vi "TEST_TRAJECTORY_EXECUTE_SWERVE.vi"(6 "EnableClosedLoop":bool=TRUE, 7 "Orientation Dmd In":dbl, 8 "Init":bool=TRUE, 9 "Reverse":bool, 10 "Follow Orientation":bool) -> (0 "AtReference":bool, 3 "Chassis Velocity Target":T2 {"vOmega" format="%10.3f"; "vY" format="%10.3f"; "vX" format="%10.3f"}, 4 "Time Offset":dbl=-1.0 format="%16.4f", 5 "Orientation Target":dbl, 11 "Gyro Heading":dbl)   [LabVIEW 2020]
uses:
  Robot Global Data.vi
  <vilib>/Rock Robotics/WPI/ThirdParty/JAS_Junk/TrajLib/Trajectory_Library.lvlib
  <vilib>/Rock Robotics/WPI/ThirdParty/JAS_Junk/TrajLib/TypeDef/CHASSIS_SPEEDS.ctl
  <vilib>/Rock Robotics/WPI/ThirdParty/JAS_Junk/TrajLib/TypeDef/TRANSLATION2D.ctl
  <vilib>/Rock Robotics/WPI/ThirdParty/JAS_Junk/TrajLib/TypeDef/ROTATION2D.ctl
  <vilib>/Rock Robotics/WPI/ThirdParty/JAS_Junk/TrajLib/TypeDef/POSE2D.ctl
  <vilib>/Rock Robotics/WPI/ThirdParty/JAS_Junk/TrajLib/TypeDef/TRAJ_STATE.ctl
panel:
  in  "Tab Control":T1(tab)
  out "OutputTRAJ_STATE":T3={"TimeSeconds"=0.0, "Velocity"=0.0, "Acceleration"=0.0, "POSE"={"TRANSLATION"={"X"=0.0, "Y"=0.0}, "ROTATION"={"VALUE"=0.0, "COS"=1.0, "SIN"=0.0}}, "Curvature"=0.0} {"POSE"."ROTATION"."SIN" format="%13.4f"; "POSE"."ROTATION"."COS" format="%13.4f"; "POSE"."ROTATION"."VALUE" format="%13.4f"; "POSE"."TRANSLATION"."Y" format="%14.3f"; "POSE"."TRANSLATION"."X" format="%14.3f"}
  in  "Step":bool
  in  "Trajectory File Name":path=path "Sample-Robot-2-Trajectory-TrajLibrary.csv"
  out "Traj File Good":bool
  out "Module Ang\nRadians":dbl
  out "Module Speed\nM/S":dbl
  in  "Run":bool
  out "Rel Odom":T4={"TRANSLATION"={"X"=0.0, "Y"=0.0}, "ROTATION"={"VALUE"=0.0, "COS"=1.0, "SIN"=0.0}} {"ROTATION"."SIN" format="%13.4f"; "ROTATION"."COS" format="%13.4f"; "ROTATION"."VALUE" format="%13.4f"; "TRANSLATION"."Y" format="%14.3f"; "TRANSLATION"."X" format="%14.3f"}
  out "Error and Corr":T7 {"Error Pose"."ROTATION"."SIN" format="%13.4f"; "Error Pose"."ROTATION"."COS" format="%13.4f"; "Error Pose"."ROTATION"."VALUE" format="%13.4f"; "Error Pose"."TRANSLATION"."Y" format="%14.3f"; "Error Pose"."TRANSLATION"."X" format="%14.3f"}
  out "Abs Odom":T4={"TRANSLATION"={"X"=0.0, "Y"=0.0}, "ROTATION"={"VALUE"=0.0, "COS"=1.0, "SIN"=0.0}} {"ROTATION"."SIN" format="%13.4f"; "ROTATION"."COS" format="%13.4f"; "ROTATION"."VALUE" format="%13.4f"; "TRANSLATION"."Y" format="%14.3f"; "TRANSLATION"."X" format="%14.3f"}
  out "Traj Err":cluster{"X":dbl, "Y":dbl, "Angle":dbl}(graph)
  out "Traj Correction":cluster{"X Corr":dbl, "Y Corr":dbl}(graph)
  out "Robot Position":cluster{dbl[], dbl[]}(graph)
  # "Module States"
  # "For now all modules use this value..."
  # "(FOR TESTING)"
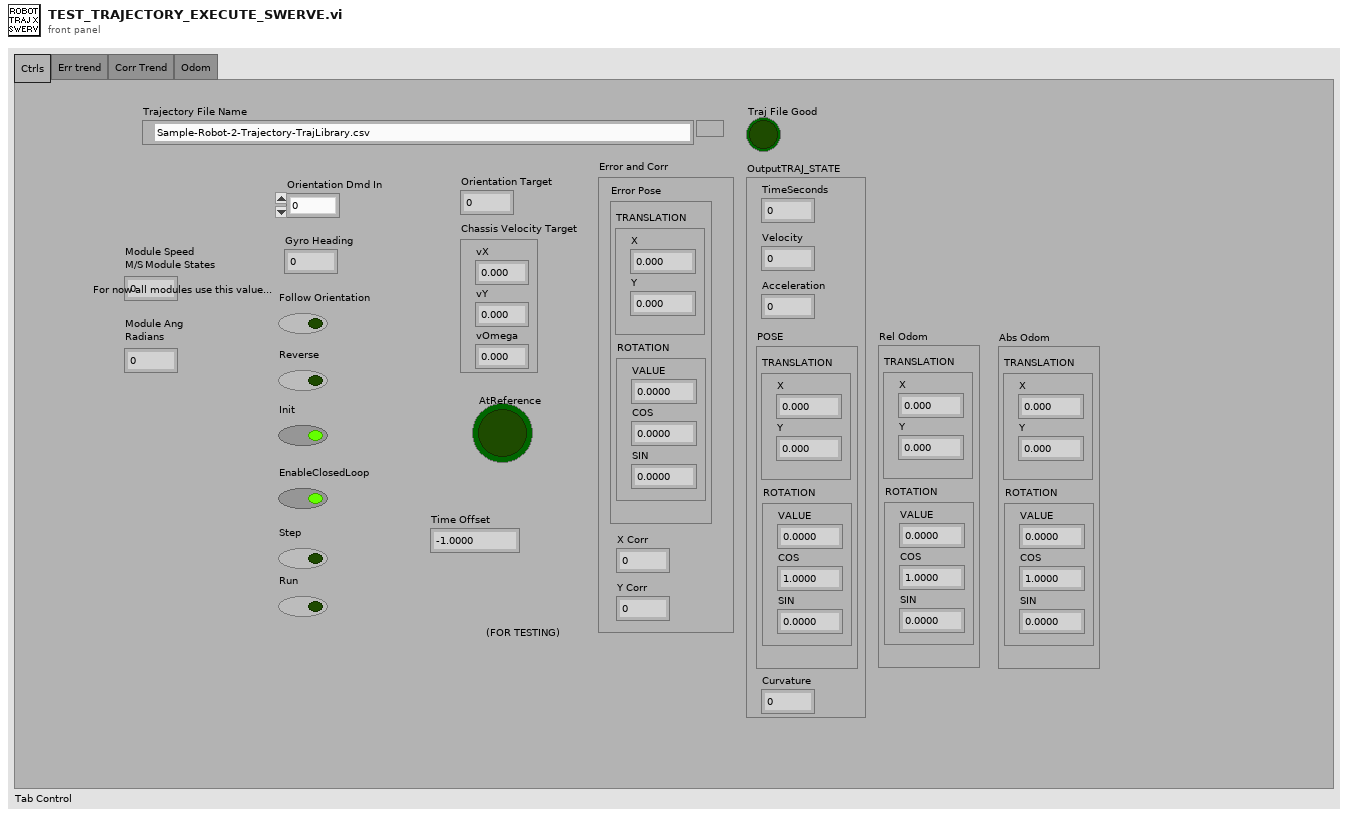
[diagram p1: front panel]
types:
  T1 = enum32{"Ctrls", "Err trend", "Corr Trend", "Odom"}
  T2 = typedef "Trajectory_Library.lvlib/CHASSIS_SPEEDS.ctl" = cluster{"vX":dbl, "vY":dbl, "vOmega":dbl}
  T3 = typedef "Trajectory_Library.lvlib/TRAJ_STATE.ctl" = cluster{"TimeSeconds":dbl, "Velocity":dbl, "Acceleration":dbl, "POSE":T4, "Curvature":dbl}
  T4 = typedef "Trajectory_Library.lvlib/POSE2D.ctl" = cluster{"TRANSLATION":T5, "ROTATION":T6}
  T5 = typedef "Trajectory_Library.lvlib/TRANSLATION2D.ctl" = cluster{"X":dbl, "Y":dbl}
  T6 = typedef "Trajectory_Library.lvlib/ROTATION2D.ctl" = cluster{"VALUE":dbl, "COS":dbl, "SIN":dbl}
  T7 = cluster{"Error Pose":T4, "X Corr":dbl, "Y Corr":dbl}
  T8 = typedef "Trajectory_Library.lvlib/SWERVE_DRIVE_ODOMETRY.ctl" = cluster{"POSE":T4, "GyroOffset":T6, "PreviousAngle":T6, "PrevModulePositions":T9[], "NumModules":i32}
  T9 = typedef "Trajectory_Library.lvlib/SWERVE_DRIVE_MODULE_POSITION.ctl" = cluster{"Distance":dbl, "Angle":T6, "P":bool}
  T10 = typedef "Trajectory_Library.lvlib/SWERVE_DRIVE_KINEMATICS.ctl" = cluster{"NumModules":i32, "InverseKinematics":T11, "ForwardKinematics":T11, "Modules":T5[], "PrevCoR":T5, "SavedModuleStates":T12[]}
  T11 = typedef "NI_Matrix.lvlib/RealMatrix.ctl" = dbl[][]
  T12 = typedef "Trajectory_Library.lvlib/SWERVE_DRIVE_MODULE_STATE.ctl" = cluster{"Speed":dbl, "Angle":T6}
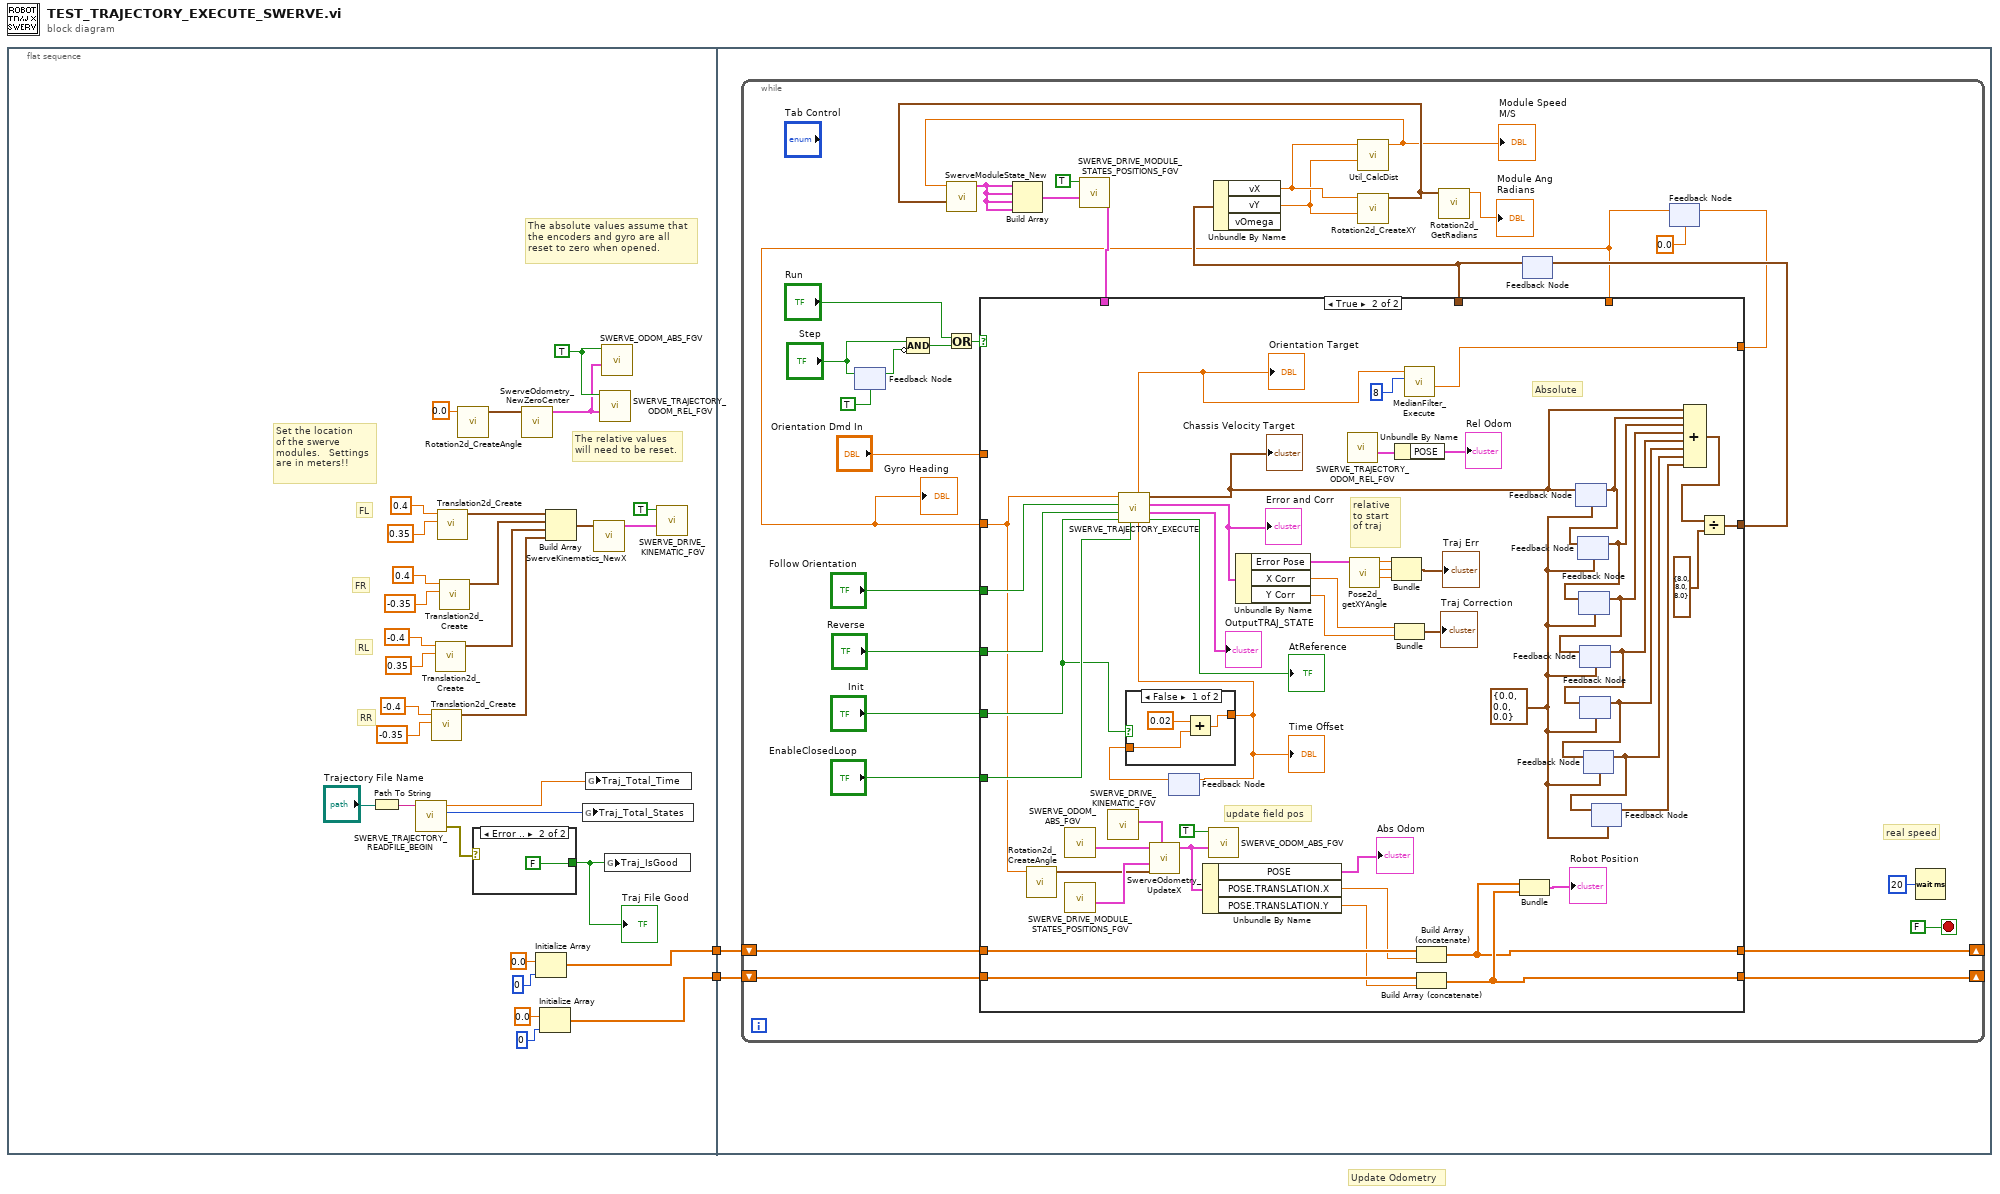
[diagram p0: block diagram]
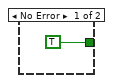
[diagram p2: hidden frame]
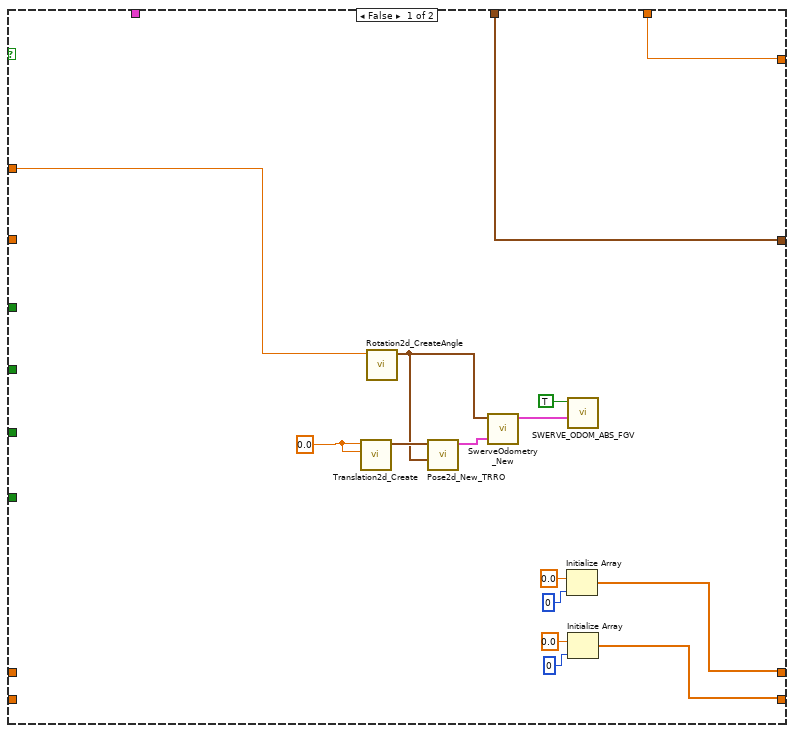
[diagram p3: hidden frame]
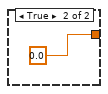
[diagram p4: hidden frame]
diagram:
  # "Update Odometry"
  n1 = flat-sequence {
    tunnel: [w8] -> w2
    tunnel: [w5] -> w1
    tunnel: w2 -> [w37]
    tunnel: w1 -> [w36]
    frame #0 {
      w4 = TRUE ("WRITE")
      # "The absolute values assume that\nthe encoders and gyro are all\nreset to zero when opened."
      # "RR"
      # "RL"
      # "FR"
      # "FL"
      # "Set the location\nof the swerve \nmodules.   Settings\nare in meters!!"
      # "The relative values\nwill need to be reset."
      n2 = Path To String(path="Trajectory File Name") -> (string=w30:string)
      n3 = call "SWERVE_TRAJECTORY_READFILE_BEGIN.vi"("Trajectory File Name"=w30) -> ("error out"=w33:errorcluster, "Trajectory Items"=w31:i32, "TotalTImeSecs"=w32:dbl)  [unwired: 8 in]
      n4 = call <vilib>:"Translation2d_Create.vi"("Y"=-0.35, "X"=-0.4) -> ("TRANSLATION"=w11:T5)  [unwired: 9 in]
      n5 = call <vilib>:"Translation2d_Create.vi"("Y"=0.35, "X"=-0.4) -> ("TRANSLATION"=w17:T5)  [unwired: 9 in]
      n6 = call <vilib>:"Translation2d_Create.vi"("Y"=0.35, "X"=0.4) -> ("TRANSLATION"=w19:T5)  [unwired: 9 in]
      n7 = call <vilib>:"Translation2d_Create.vi"("Y"=-0.35, "X"=0.4) -> ("TRANSLATION"=w18:T5)  [unwired: 9 in]
      n8 = call <vilib>:"Rotation2d_CreateAngle.vi"("Angle"=0.0) -> ("ROTATION"=w26:T6)  [unwired: 10 in]
      n9 = case shown="Error .." w33 {
        tunnel: [TRUE FALSE] -> w28
        frame No Error {
        }
        frame Error {
        }
      }
      "Traj File Good" <- w28
      n10 = call <vilib>:"SwerveOdometry_NewZeroCenter.vi"("gyroAngle"=w26) -> ("SWERVE_DRIVE_ODOMETRY"=w3:T8)  [unwired: 10 in]
      n11 = Initialize Array(0.0 ("element"), 0 ("dimension size")) -> (w8:dbl[])
      n12 = Initialize Array(0.0 ("element"), 0 ("dimension size")) -> (w5:dbl[])
      n13 = Build Array(w19, w18, w17, w11) -> (w16:T5[])
      n14 = global write "Robot Global Data.vi" "Traj_Total_States"(w31) -> ()
      n15 = global write "Robot Global Data.vi" "Traj_Total_Time"(w32) -> ()
      n16 = call <vilib>:"SwerveKinematics_NewX.vi"("Wheels"=w16) -> ("SWERVE_DRIVE_KINEMATICS"=w14:T10)  [unwired: 10 in]
      n17 = call "SWERVE_TRAJECTORY_ODOM_REL_FGV.vi"("in SWERVE_DRIVE_ODOMETRY"=w3, "WRITE"=w4) -> ()  [unwired: 9 in, 1 out]
      n18 = call "SWERVE_ODOM_ABS_FGV.vi"("in SWERVE_DRIVE_ODOMETRY"=w3, "WRITE"=w4) -> ()  [unwired: 9 in, 1 out]
      n19 = global write "Robot Global Data.vi" "Traj_IsGood"(w28) -> ()
      n20 = call "SWERVE_DRIVE_KINEMATIC_FGV.vi"("in SWERVE_DRIVE_KINEMATICS"=w14, "WRITE"=TRUE) -> ()  [unwired: 9 in, 1 out]
    }
    frame #1 {
      n21 = while {
        shift-right: [w38] -> _
        shift-left: w37 -> [w41]
        shift-right: [w39] -> _
        shift-left: w36 -> [w40]
        stop <- FALSE stop-if-true
        # "real speed"
        n22 = feedback #1(TRUE ("Step")) -> (w65:bool)
        n23 = feedback-in #1("Step") -> ()
        n24 = Compound Arithmetic op=AND("Step", invert w65) -> (w48:bool)
        n25 = Or(x="Run", y=w48) -> (x .or. y?=w47:bool)
        n26 = feedback #2() -> (w54:T2)  [unwired: 1 in]
        n27 = Unbundle By Name(w54) -> ("vX"=w53:dbl, "vY"=w52:dbl)  [unwired: 1 out]
        n28 = call <vilib>:"Util_CalcDist.vi"("Y"=w52, "X"=w53) -> ("DIST"=w49:dbl)  [unwired: 9 in]
        "Module Speed\nM/S" <- w49
        n29 = call <vilib>:"Rotation2d_CreateXY.vi"("Y or sine"=w52, "X or  cosine"=w53) -> ("ROTATION"=w51:T6)  [unwired: 9 in]
        n30 = call <vilib>:"SwerveModuleState_New.vi"("ROTATION"=w51, "Speed"=w49) -> ("SWERVE_DRIVE_MODULE_STATE"=w57:T12)  [unwired: 9 in]
        n31 = Build Array(w57, w57, w57, w57) -> (w58:T12[])
        n32 = call "SWERVE_DRIVE_MODULE_STATES_POSITIONS_FGV.vi"("in Current Module States"=w58, "WRITE"=TRUE) -> ("out Current Module States"=w59:T12[])  [unwired: 8 in, 1 out]
        n33 = call <vilib>:"Rotation2d_GetRadians.vi"("in ROTATION"=w51) -> ("AngleRadians"=→"Module Ang\nRadians":dbl)  [unwired: 10 in]
        n34 = feedback #3(0.0 ("MedianValue")) -> (w43:dbl)
        "Gyro Heading" <- w43
        n35 = case shown="True" w47 {
          tunnel: w43 -> [_ w85]
          tunnel: "Follow Orientation" -> [_ w132]
          tunnel: "Reverse" -> [_ w131]
          tunnel: "Init" -> [_ w126]
          tunnel: "EnableClosedLoop" -> [_ w130]
          tunnel: "Orientation Dmd In" -> [w74 _]
          tunnel: w59 -> [_ _]
          tunnel: [w83 w113] -> w55
          tunnel: w54 -> [w83 _]
          tunnel: [w82 w106] -> w45
          tunnel: w43 -> [w82 _]
          tunnel: w41 -> [_ w97]
          tunnel: w40 -> [_ w98]
          tunnel: [w79 w95] -> w39
          tunnel: [w76 w94] -> w38
          frame False {
            w72 = 0.0 ("X")
            n36 = call <vilib>:"Translation2d_Create.vi"("Y"=w72, "X"=w72) -> ("TRANSLATION"=w73:T5)  [unwired: 9 in]
            n37 = call <vilib>:"Rotation2d_CreateAngle.vi"("Angle"=w74) -> ("ROTATION"=w71:T6)  [unwired: 10 in]
            n38 = call <vilib>:"Pose2d_New_TRRO.vi"("ROTATION"=w71, "TRANSLATION"=w73) -> ("outPOSE"=w70:T4)  [unwired: 9 in]
            n39 = call <vilib>:"SwerveOdometry_New.vi"("InitialPose"=w70, "gyroAngle"=w71) -> ("SWERVE_DRIVE_ODOMETRY"=w69:T8)  [unwired: 9 in]
            n40 = Initialize Array(0.0 ("element"), 0 ("dimension size")) -> (w76:dbl[])
            n41 = call "SWERVE_ODOM_ABS_FGV.vi"("in SWERVE_DRIVE_ODOMETRY"=w69, "WRITE"=TRUE) -> ()  [unwired: 9 in, 1 out]
            n42 = Initialize Array(0.0 ("element"), 0 ("dimension size")) -> (w79:dbl[])
          }
          frame True {
            w124 = T2 {"vX"=0.0, "vY"=0.0, "vOmega"=0.0} ("Chassis Velocity Target")
            # "update field pos"
            # "Absolute"
            # "relative to start of traj"
            n43 = call <vilib>:"Rotation2d_CreateAngle.vi"("Angle"=w85) -> ("ROTATION"=w90:T6)  [unwired: 10 in]
            n44 = call "SWERVE_ODOM_ABS_FGV.vi"() -> ("out SWERVE_DRIVE_ODOMETRY"=w93:T8)  [unwired: 11 in]
            n45 = call "SWERVE_DRIVE_MODULE_STATES_POSITIONS_FGV.vi"() -> ("out Current Module States"=w91:T12[])  [unwired: 10 in, 1 out]
            n46 = call "SWERVE_DRIVE_KINEMATIC_FGV.vi"() -> ("out SWERVE_DRIVE_KINEMATICS"=w92:T10)  [unwired: 11 in]
            n47 = call <vilib>:"SwerveOdometry_UpdateX.vi"(7:w92, "module Positions"=w90, "gyroAngle"=w91, "SWERVE_DRIVE_KINEMATICS"=w93) -> ("out SWERVE_DRIVE_ODOMETRY"=w88:T8)  [unwired: 5 in, 2 out]
            n48 = feedback #4() -> (w127:dbl)  [unwired: 1 in]
            n49 = case shown="False" w126 {
              tunnel: [w135 0.0] -> w125
              tunnel: w127 -> [w133 _]
              frame False {
                n50 = Add(x=0.02, y=w133) -> (x+y=w135:dbl)
              }
              frame True {
              }
            }
            "Time Offset" <- w125
            n51 = call "SWERVE_TRAJECTORY_EXECUTE.vi"("Time Offset"=w125, "EnableClosedLoop"=w130, "Init"=w126, "Reverse"=w131, "Follow Orientation"=w132, "Gyro Heading\nRAD"=w85) -> ("AtReference"=→"AtReference":bool, "OutputTRAJ_STATE"=→"OutputTRAJ_STATE":T3, "Error and Corr"=w105:T7, "Chassis Velocity Target"=w123:T2, "Orientation Target"=w108:dbl)  [unwired: 1 in]
            "Orientation Target" <- w108
            "Chassis Velocity Target" <- w123
            "Error and Corr" <- w105
            n52 = feedback-in #4(w125) -> ()
            n53 = Unbundle By Name(w88) -> ("POSE"=→"Abs Odom":T4, "POSE.TRANSLATION.X"=w87:dbl, "POSE.TRANSLATION.Y"=w86:dbl)
            n54 = call "SWERVE_ODOM_ABS_FGV.vi"("in SWERVE_DRIVE_ODOMETRY"=w88, "WRITE"=TRUE) -> ()  [unwired: 9 in, 1 out]
            n55 = Unbundle By Name(w105) -> ("Error Pose"=w104:T4, "X Corr"=w103:dbl, "Y Corr"=w102:dbl)
            n56 = call "SWERVE_TRAJECTORY_ODOM_REL_FGV.vi"() -> ("out SWERVE_DRIVE_ODOMETRY"=w99:T8)  [unwired: 11 in]
            n57 = call <vilib>:"Pose2d_getXYAngle.vi"("in POSE"=w104) -> ("Angle"=w109:dbl, "Y"=w110:dbl, "X"=w111:dbl)  [unwired: 8 in]
            n58 = Bundle("X"=w111, "Y"=w110, "Angle"=w109) -> (→"Traj Err":cluster{"X":dbl, "Y":dbl, "Angle":dbl})  [unwired: 1 in]
            n59 = Unbundle By Name(w99) -> ("POSE"=→"Rel Odom":T4)
            n60 = Bundle("X Corr"=w103, "Y Corr"=w102) -> (→"Traj Correction":cluster{"X Corr":dbl, "Y Corr":dbl})  [unwired: 1 in]
            n61 = call <vilib>:"MedianFilter_Execute.vi"("Samples"=8, "Input Value"=w108) -> ("MedianValue"=w106:dbl)  [unwired: 8 in, 1 out]
            n62 = Build Array (concatenate)(w97, w87) -> (w94:dbl[])
            n63 = Build Array (concatenate)(w98, w86) -> (w95:dbl[])
            n64 = Bundle(w94, w95) -> (→"Robot Position":cluster{dbl[], dbl[]})  [unwired: 1 in]
            n65 = feedback-in #5(w123) -> ()
            n66 = feedback #5(w124) -> (w122:T2)
            n67 = feedback #6(w124) -> (w121:T2)
            n68 = feedback-in #6(w122) -> ()
            n69 = feedback #7(w124) -> (w120:T2)
            n70 = feedback-in #7(w121) -> ()
            n71 = feedback #8(w124) -> (w119:T2)
            n72 = feedback-in #8(w120) -> ()
            n73 = feedback #9(w124) -> (w118:T2)
            n74 = feedback-in #9(w119) -> ()
            n75 = feedback #10(w124) -> (w117:T2)
            n76 = feedback-in #10(w118) -> ()
            n77 = feedback #11(w124) -> (w116:T2)
            n78 = feedback-in #11(w117) -> ()
            n79 = Compound Arithmetic op=ADD(w123, w122, w121, w120, w119, w118, w117, w116) -> (w115:T2)
            n80 = Divide(x=w115, y=T2 {"vX"=8.0, "vY"=8.0, "vOmega"=8.0}) -> (x/y=w113:T2)
          }
        }
        n81 = feedback-in #2(w55) -> ()
        n82 = feedback-in #3(w45) -> ()
        n83 = Wait (ms)(milliseconds to wait=u32 20) -> ()  [unwired: 1 out]
      }
    }
  }
